vi "Inverse Kinematics Old.vi"() -> ()   [LabVIEW 2020]
panel:
  out "T4":dbl
  out "T3":dbl
  out "T2":dbl
  out "T1":dbl
  out "V4":dbl
  out "V3":dbl
  out "V2":dbl
  out "V1":dbl
  in  "r4y":dbl
  in  "r3y":dbl
  in  "r2y":dbl
  in  "r1y":dbl
  in  "r4x":dbl
  in  "r3x":dbl
  in  "r2x":dbl
  in  "r1x":dbl
  in  "Vx":dbl
  in  "Vy":dbl
  in  "w //omega":dbl
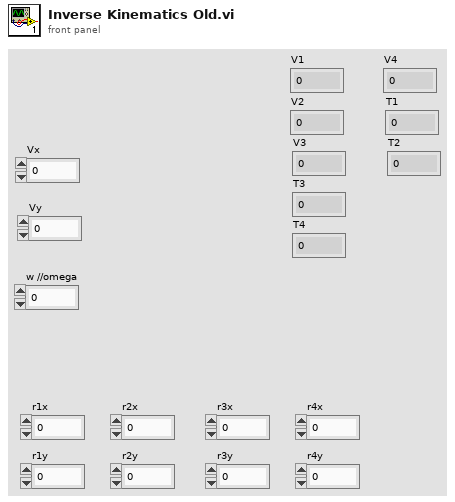
[diagram p1: front panel]
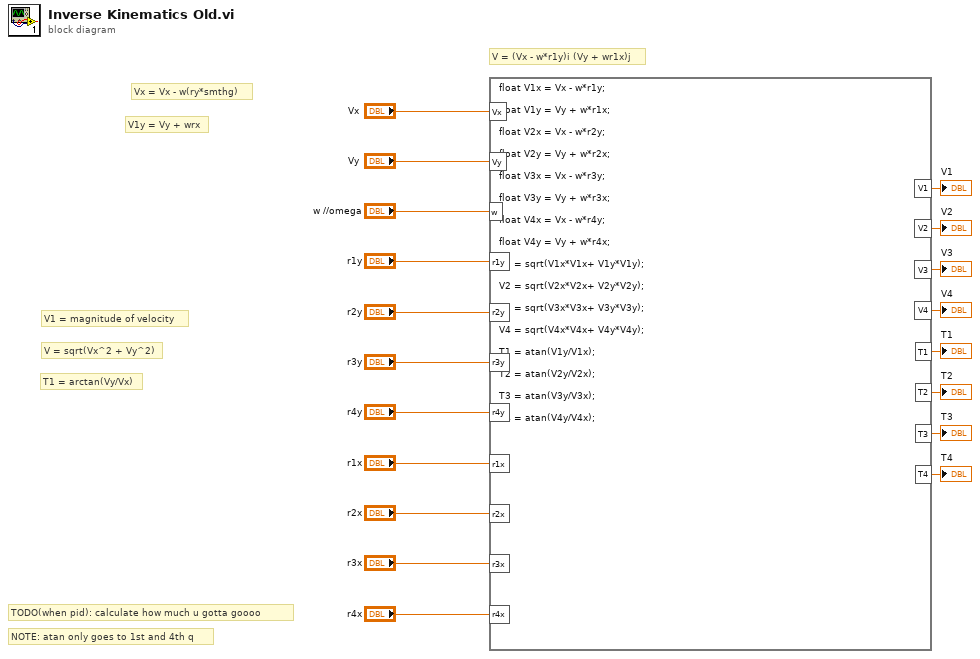
[diagram p0: block diagram]
diagram:
  # "NOTE: atan only goes to 1st and 4th q"
  # "T1 = arctan(Vy/Vx)"
  # "V1 = magnitude of velocity"
  # "V = sqrt(Vx^2 + Vy^2)"
  # "TODO(when pid): calculate how much u gotta goooo"
  # "V1y = Vy + wrx"
  # "Vx = Vx - w(ry*smthg)"
  # "V = (Vx - w*r1y)i (Vy + wr1x)j"
  n1 = formula code="float V1x = Vx - w*r1y; \n\nfloat V1y = Vy + w*r1x;\n\nfloat V2x = Vx - w*r2y; \n\nfloat V2y = Vy + w*r2x;\n\nfloat V3x = Vx - w*r3y; \n\nfloat V3y = Vy + w*r3x;\n\nfloat V4x = Vx - w*r4y; \n\nfloat V4y = Vy + w*r4x;\n\nV1 = sqrt(V1x*V1x+ V1y*V1y); \n\nV2 = sqrt(V2x*V2x+ V2y*V2y); \n\nV3 = sqrt(V3x*V3x+ V3y*V3y); \n\nV4 = sqrt(V4x*V4x+ V4y*V4y); \n\nT1 = atan(V1y/V1x);\n\nT2 = atan(V2y/V2x);\n\nT3 = atan(V3y/V3x);\n\nT4 = atan(V4y/V4x);"("w"="w //omega", "Vy"="Vy", "r3y"="r3y", "r2y"="r2y", "r1x"="r1x", "r2x"="r2x", "r3x"="r3x", "r4x"="r4x", "r1y"="r1y", "r4y"="r4y", "Vx"="Vx") -> ("V1"=→"V1":dbl, "V2"=→"V2":dbl, "V3"=→"V3":dbl, "V4"=→"V4":dbl, "T1"=→"T1":dbl, "T2"=→"T2":dbl, "T3"=→"T3":dbl, "T4"=→"T4":dbl)
